vi "labview2tikz_XY.vi"(8 "error in (no error)":errorcluster, 10 "file (use dialog)":path, 11 "XY Graph 2":refnum<vi>) -> (0 "error out":errorcluster, 3 "result string":string)   [LabVIEW 2012]
uses:
  pgfPlotPlot_tdef.ctl
  pgfPlotAxis_tdef.ctl
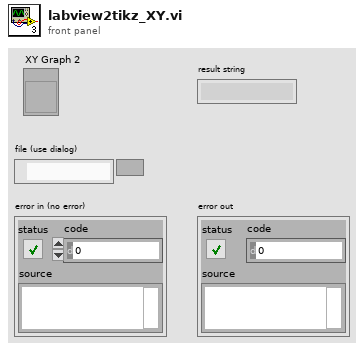
[diagram p1: front panel]
types:
  T1 = typedef "pgfPlotAxis_tdef.ctl" = cluster{"xmin":dbl, "xmax":dbl, "ymin":dbl, "ymax":dbl, "xLabel":string, "yLabel":string}
  T2 = typedef "pgfPlotPlot_tdef.ctl" = cluster{"LineStyle":u8, "LineWidth":u8, "PlotColor":u32, "Marker":u8, "PlotName":string, "x values":dbl[], "y values":dbl[]}
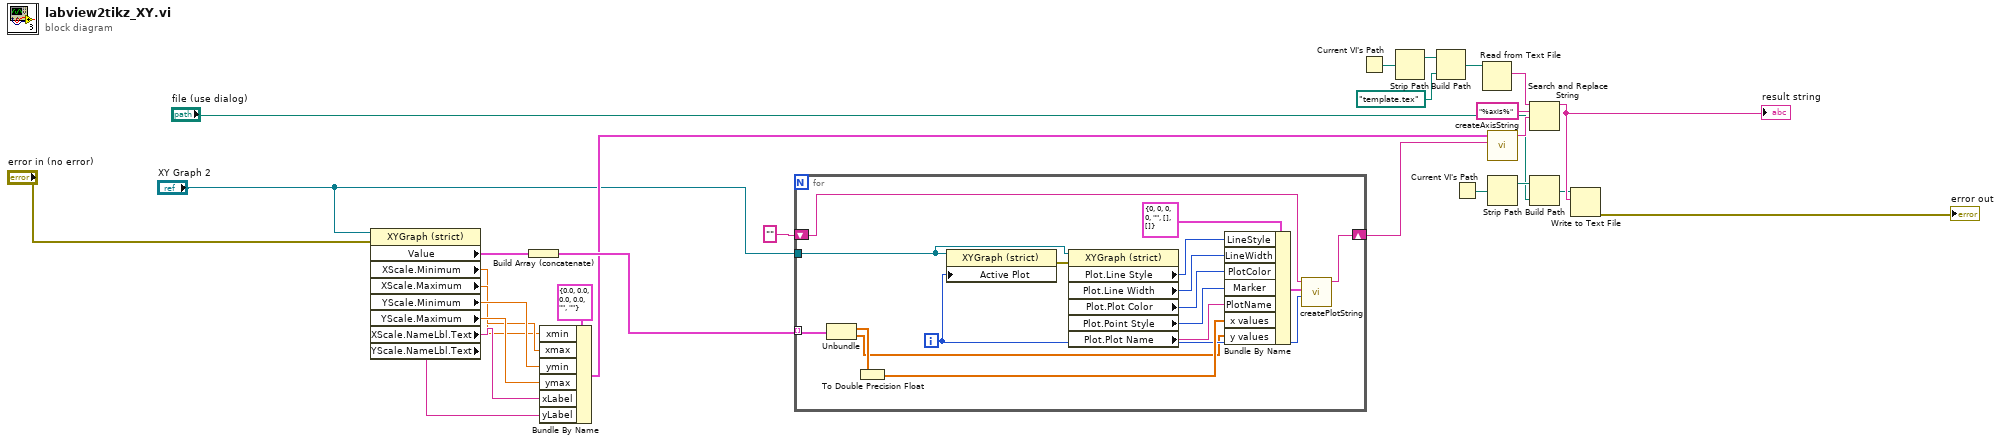
[diagram p0: block diagram]
diagram:
  n1 = property class="XYGraph (strict)"(reference="XY Graph 2", error in="error in (no error)") -> ("Value"=w10:cluster{"Array":dbl[], "Array 3":dbl[]}[], "XScale.Minimum"=w14:dbl, "XScale.Maximum"=w15:dbl, "YScale.Minimum"=w16:dbl, "YScale.Maximum"=w17:dbl, "XScale.NameLbl.Text"=w18:string, "YScale.NameLbl.Text"=w19:string)  [unwired: 2 out]
  n2 = Build Array (concatenate)(w10) -> (w27:cluster{"Array":dbl[], "Array 3":dbl[]}[])
  n3 = Bundle By Name(cluster=T1 {"xmin"=0.0, "xmax"=0.0, "ymin"=0.0, "ymax"=0.0, "xLabel"="", "yLabel"=""} ("Input"), "xmin"=w14, "xmax"=w15, "ymin"=w16, "ymax"=w17, "xLabel"=w18, "yLabel"=w19) -> (w20:T1)
  n4 = for {
    tunnel: "XY Graph 2" -> [w43]
    tunnel: w27 -> [w30] mode=indexing
    shift-right: [w41] -> w23
    shift-left: "" -> [w32]
    i -> [w31]
    n5 = Unbundle(w30) -> ("Array"=w29:dbl[], "Array 3"=w28:dbl[])
    n6 = To Double Precision Float(number=w29) -> (double precision float=w33:dbl[])
    n7 = property class="XYGraph (strict)"(reference=w43, "Active Plot"=w31) -> (error out=w42:errorcluster)  [unwired: 1 in, 1 out]
    n8 = property class="XYGraph (strict)"(reference=w43, error in=w42) -> ("Plot.Line Style"=w39:u8, "Plot.Line Width"=w38:u8, "Plot.Plot Color"=w34:u32, "Plot.Point Style"=w37:u8, "Plot.Plot Name"=w36:string)  [unwired: 2 out]
    n9 = Bundle By Name(cluster=T2 {"LineStyle"=0, "LineWidth"=0, "PlotColor"=0, "Marker"=0, "PlotName"="", "x values"=[], "y values"=[]}, "LineStyle"=w39, "LineWidth"=w38, "PlotColor"=w34, "Marker"=w37, "PlotName"=w36, "x values"=w33, "y values"=w28) -> (w35:T2)
    n10 = call "createPlotString.vi"("current plot number"=w31, "Plot Data"=w35, "plot string in"=w32) -> ("plot string out"=w41:string)  [unwired: 8 in]
  }
  n11 = Current VI's Path() -> (path=w2:path)
  n12 = Strip Path(path=w2) -> (stripped path=w3:path)  [unwired: 1 out]
  n13 = Build Path(base path=w3, name or relative path=path "template.tex" ("file (use dialog)")) -> (appended path=w5:path)
  n14 = Current VI's Path() -> (path=w8:path)
  n15 = Read from Text File(file (use dialog)=w5) -> (text=w12:string)  [unwired: 3 in, 3 out]
  n16 = call "createAxisString.vi"("PlotsString"=w23, "Input Data"=w20) -> ("AxisString"=w22:string)  [unwired: 9 in]
  n17 = Strip Path(path=w8) -> (stripped path=w7:path)  [unwired: 1 out]
  n18 = Search and Replace String(input string=w12, search string="%axis%", replace string=w22) -> (result string=w24:string)  [unwired: 5 in, 3 out]
  "result string" <- w24
  n19 = Build Path(base path=w7, name or relative path="file (use dialog)") -> (appended path=w9:path)
  n20 = Write to Text File(file (use dialog)=w9, text=w24) -> (error out=→"error out":errorcluster)  [unwired: 2 in, 2 out]
